vi "Refresh UI.vi"(8 "error in (no error)":errorcluster, 11 "Configuration UI in":refnum<class "Configuration UI.lvclass">) -> (0 "error out":errorcluster, 3 "Configuration UI out":refnum<class "Configuration UI.lvclass">)   [LabVIEW 2019, in "Configuration UI.lvlib" / "Configuration UI.lvclass"]
doc: "Reload the configuration file (ensuring the GUI matches the config.ini file data)\n\nRead the complete list of devices defined in config.ini and update the Instruments listbox \n- This allows the user to select defined instruments from the listbox\n\nIf an active device is already selected, make sure that item is selected in the listbox."
uses:
  Project/Configuration UI.lvclass
  Project/Configuration UI.lvclass/Configuration UI.ctl
  builds/Tools/Config.lvlibp/Config.lvclass
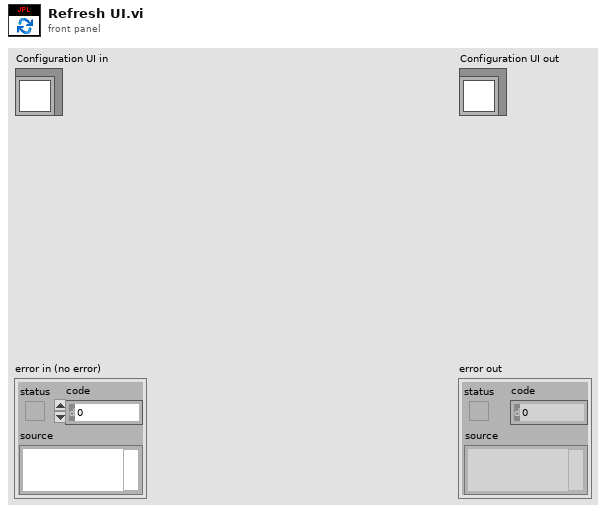
[diagram p1: front panel]
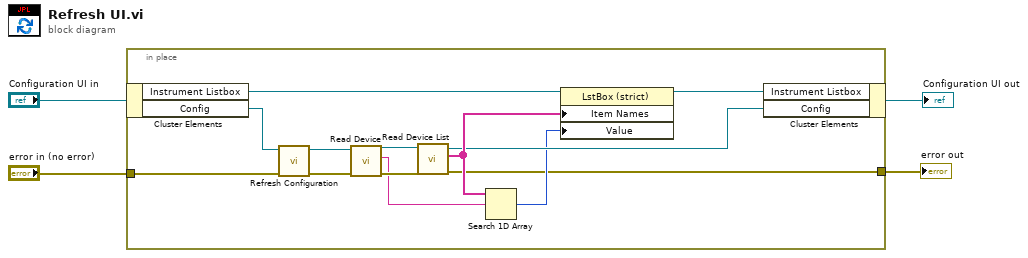
[diagram p0: block diagram]
diagram:
  n1 = in-place {
    in-place-border: "error in (no error)" -> [w16]
    in-place-border: [w5] -> w1
    n2 = in-place-cluster #1("Configuration UI in") -> ("Instrument Listbox"=w11:refnum<vi>, "Config"=w17:refnum<class "Config.lvclass">)
    n3 = call "Refresh Configuration.vi"("error in"=w16, "Config in"=w17) -> ("error out"=w14:errorcluster, "Config out"=w15:refnum<class "Config.lvclass">)  [unwired: 8 in]
    n4 = call "Read Device.vi"("error in"=w14, "Config in"=w15) -> ("error out"=w12:errorcluster, "Device"=w10:string, "Config out"=w13:refnum<class "Config.lvclass">)  [unwired: 7 in]
    n5 = call "Read Device List.vi"("error in"=w12, "Config in"=w13) -> ("error out"=w5:errorcluster, "Device List"=w9:string[], "Config out"=w7:refnum<class "Config.lvclass">)  [unwired: 7 in]
    n6 = Search 1D Array(1D array=w9, element=w10) -> (index of element=w6:i32)  [unwired: 1 in]
    n7 = property class="LstBox (strict)"(reference=w11, "Item Names"=w9, "Value"=w6) -> (reference out=w8:refnum<vi>)  [unwired: 1 in, 1 out]
    n8 = in-place-cluster #1("Instrument Listbox"=w8, "Config"=w7) -> (→"Configuration UI out":refnum<class "Configuration UI.lvclass">)
  }
  "error out" <- w1
